vi "Unflatten Pixmap.vi"(10 "image data":T1) -> (0 "1-bit pixmap":bool[][](array[boolean]), 1 "4-bit pixmap":u8[][](array[numeric]), 2 "8-bit pixmap":u8[][](array[numeric]), 3 "24-bit pixmap":u32[][](array[numeric]) format="%x", 4 "colors":u32[](array[numeric]), 5 "top left":cluster{"x":i16, "y":i16}, 6 "mask":u8[](array[numeric]))   [LabVIEW 2017]
doc: "Converts a cluster of image data into a 2D array."
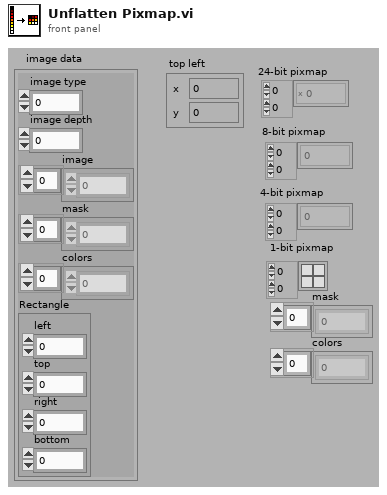
[diagram p1: front panel]
types:
  T1 = cluster{"image type":i32, "image depth":i32, "image":u8[], "mask":u8[], "colors":u32[], "Rectangle":cluster{"left":i16, "top":i16, "right":i16, "bottom":i16}}
  T2 = cluster{"left":i16, "top":i16, "right":i16, "bottom":i16}
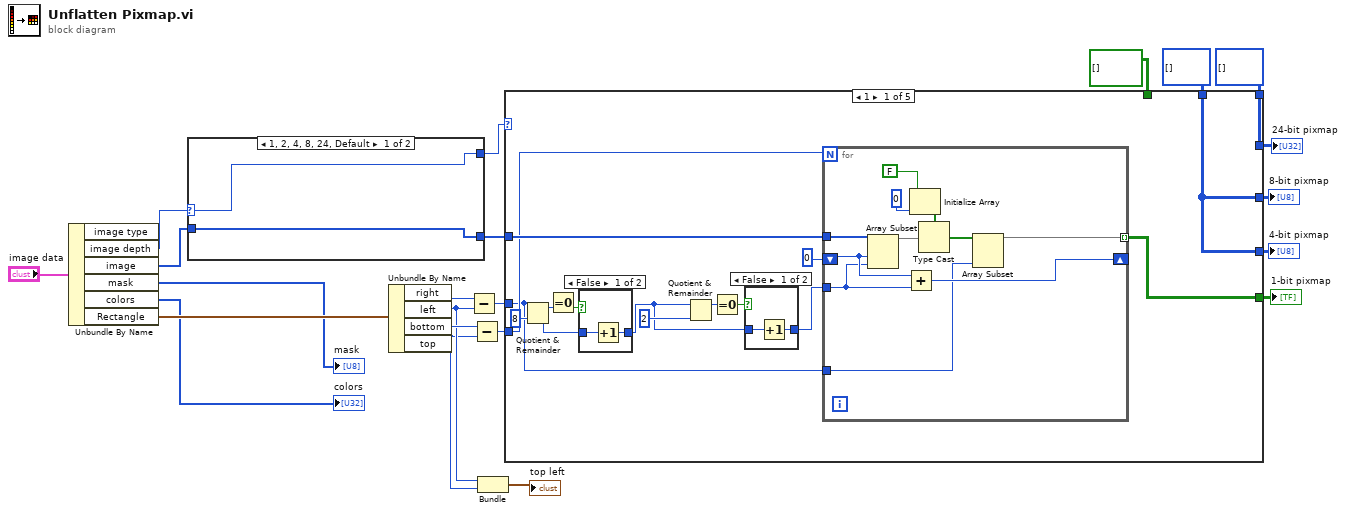
[diagram p0: block diagram]
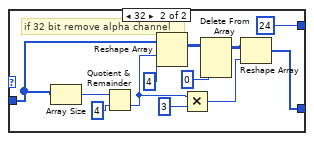
[diagram p2: hidden frame]
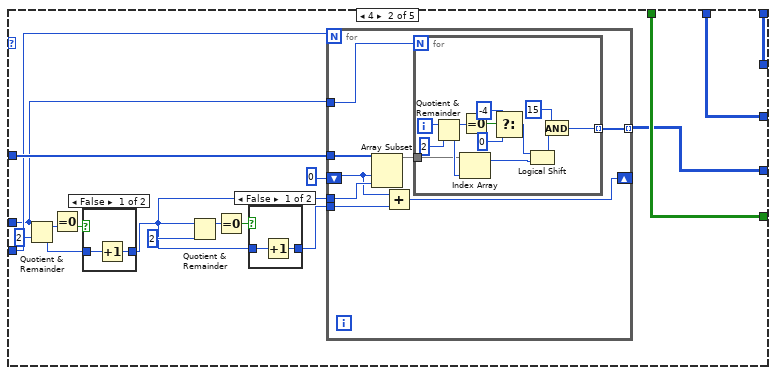
[diagram p5: hidden frame]
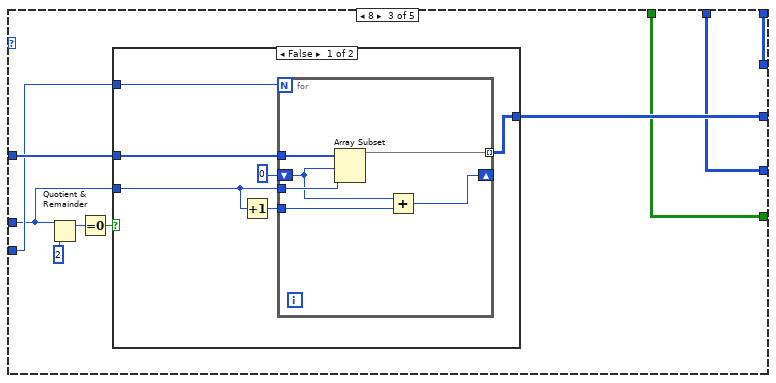
[diagram p8: hidden frame]
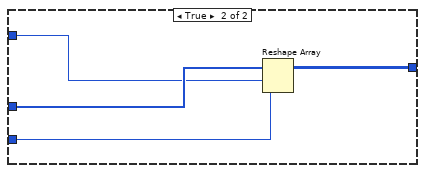
[diagram p9: hidden frame]
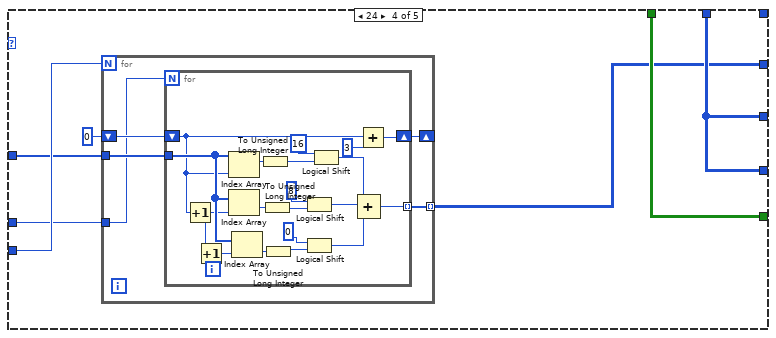
[diagram p10: hidden frame]
diagram:
  n1 = Unbundle By Name("image data") -> ("image depth"=w1:i32, "image"=w4:u8[], "mask"=→"mask":u8[], "colors"=→"colors":u32[], "Rectangle"=w7:T2)  [unwired: 1 out]
  n2 = case shown="1, 2, 4, 8, 24, Default" w1 {
    selector: w1 -> [w24 _]
    tunnel: [w24 24] -> w2
    tunnel: w4 -> [w23 w35]
    tunnel: [w23 w26] -> w3
    frame 1, 2, 4, 8, 24, Default {
    }
    frame 32 {
      # "if 32 bit remove alpha channel"
      n3 = Array Size(array=w35) -> (size(s)=w34:i32)
      n4 = Quotient & Remainder(x=w34, y=4) -> (floor(x/y)=w30:i32)  [unwired: 1 out]
      n5 = Reshape Array(w35, w30, 4 ("dimension size")) -> (w32:u8[][])
      n6 = Multiply(x=w30, y=3) -> (x*y=w28:i32)
      n7 = Delete From Array(array=w32, index (col)=0 ("dimension size")) -> (array with subset deleted=w27:u8[][])  [unwired: 2 in, 1 out]
      n8 = Reshape Array(w27, w28) -> (w26:u8[])
    }
  }
  n9 = Unbundle By Name(w7) -> ("right"=w22:i16, "left"=w10:i16, "bottom"=w21:i16, "top"=w9:i16)
  n10 = Subtract(x=w22, y=w10) -> (x-y=w20:i16)
  n11 = Subtract(x=w21, y=w9) -> (x-y=w19:i16)
  n12 = Bundle("left"=w10, "top"=w9) -> (→"top left":cluster{"left":i16, "top":i16})  [unwired: 1 in]
  n13 = case shown="1" w2 {
    tunnel: w3 -> [w52 w86 w121 w142 _]
    tunnel: w20 -> [w39 w72 w118 w143 _]
    tunnel: w19 -> [w44 w78 w119 w144 _]
    tunnel: [w47 w71 w114 w146 w172] -> w18
    tunnel: u8[][] [] ("4-bit pixmap") -> [w46 w80 w115 w145 w171]
    tunnel: [w46 w70 w115 w145 w171] -> w16
    tunnel: bool[][] [] ("1-bit pixmap") -> [_ w71 w114 w146 w172]
    tunnel: [w46 w80 w120 w145 w171] -> w14
    tunnel: [w45 w79 w116 w141 w173] -> w13
    tunnel: u32[][] [] ("24-bit pixmap") -> [w45 w79 w116 _ w173]
    frame 1 {
      n14 = Quotient & Remainder(x=w39, y=i16 8) -> (x-y*floor(x/y)=w42:i16, floor(x/y)=w40:i16)
      n15 = Equal To 0?(x=w42) -> (x = 0?=w41:bool)
      n16 = case shown="False" w41 {
        tunnel: w40 -> [w54 w55]
        tunnel: [w53 w55] -> w38
        frame False {
          n17 = Increment(x=w54) -> (x+1=w53:i16)
        }
        frame True {
        }
      }
      n18 = Quotient & Remainder(x=w38, y=2) -> (x-y*floor(x/y)=w50:i32)  [unwired: 1 out]
      n19 = Equal To 0?(x=w50) -> (x = 0?=w49:bool)
      n20 = case shown="False" w49 {
        tunnel: w38 -> [w57 w58]
        tunnel: [w56 w58] -> w37
        frame False {
          n21 = Increment(x=w57) -> (x+1=w56:i16)
        }
        frame True {
        }
      }
      n22 = for {
        N: w44 -> [_]
        tunnel: w52 -> [w69]
        shift-right: [w64] -> _
        shift-left: 0 -> [w68]
        tunnel: w37 -> [w59]
        tunnel: [w61] -> w47 mode=indexing
        tunnel: w39 -> [w62]
        n23 = Array Subset(array=w69, index=w68, length=w59) -> (w60:u8[])
        n24 = Add(x=w68, y=w59) -> (x+y=w64:i32)
        n25 = Initialize Array(FALSE, i16 0) -> (w67:bool[])
        n26 = Type Cast(type=w67, x=w60) -> (*(type *) &x=w63:bool[])
        n27 = Array Subset(array=w63, length=w62) -> (w61:bool[])  [unwired: 1 in]
      }
    }
    frame 4 {
      n28 = Quotient & Remainder(x=w72, y=i16 2) -> (x-y*floor(x/y)=w76:i16, floor(x/y)=w74:i16)
      n29 = Equal To 0?(x=w76) -> (x = 0?=w75:bool)
      n30 = case shown="False" w75 {
        tunnel: w74 -> [w88 w89]
        tunnel: [w87 w89] -> w73
        frame False {
          n31 = Increment(x=w88) -> (x+1=w87:i16)
        }
        frame True {
        }
      }
      n32 = Quotient & Remainder(x=w73, y=2) -> (x-y*floor(x/y)=w84:i32)  [unwired: 1 out]
      n33 = Equal To 0?(x=w84) -> (x = 0?=w83:bool)
      n34 = case shown="False" w83 {
        tunnel: w73 -> [w91 w92]
        tunnel: [w90 w92] -> w81
        frame False {
          n35 = Increment(x=w91) -> (x+1=w90:i16)
        }
        frame True {
        }
      }
      n36 = for {
        N: w78 -> [_]
        tunnel: w86 -> [w100]
        shift-right: [w96] -> _
        shift-left: 0 -> [w98]
        tunnel: w73 -> [w99]
        tunnel: w81 -> [w97]
        tunnel: w72 -> [w93]
        tunnel: [w94] -> w70 mode=indexing
        n37 = Array Subset(array=w100, index=w98, length=w99) -> (w95:u8[])
        n38 = Add(x=w98, y=w97) -> (x+y=w96:i32)
        n39 = for {
          N: w93 -> [_]
          tunnel: w95 -> [w107]
          tunnel: [w108] -> w94 mode=indexing
          i -> [w112]
          n40 = Quotient & Remainder(x=w112, y=2) -> (x-y*floor(x/y)=w105:i32, floor(x/y)=w111:i32)
          n41 = Index Array(array=w107, index=w111) -> (element=w106:u8)
          n42 = Equal To 0?(x=w105) -> (x = 0?=w104:bool)
          n43 = Select(t=i8 -4, s=w104, f=i8 0) -> (s? t:f=w101:i8)
          n44 = Logical Shift(y=w101, x=w106) -> (x << y=w109:u8)
          n45 = And(x=u8 15, y=w109) -> (x .and. y?=w108:u8)
        }
      }
    }
    frame 8 {
      n46 = Quotient & Remainder(x=w118, y=2) -> (x-y*floor(x/y)=w122:i32)  [unwired: 1 out]
      n47 = Equal To 0?(x=w122) -> (x = 0?=w117:bool)
      n48 = case shown="False" w117 {
        tunnel: w121 -> [w129 w138]
        tunnel: [w126 w139] -> w120
        tunnel: w119 -> [w128 w137]
        tunnel: w118 -> [w125 w136]
        frame False {
          n49 = Increment(x=w125) -> (x+1=w124:i16)
          n50 = for {
            N: w128 -> [_]
            tunnel: w129 -> [w135]
            shift-right: [w132] -> _
            shift-left: 0 -> [w133]
            tunnel: w125 -> [w134]
            tunnel: [w131] -> w126 mode=indexing
            tunnel: w124 -> [w130]
            n51 = Array Subset(array=w135, index=w133, length=w134) -> (w131:u8[])
            n52 = Add(x=w133, y=w130) -> (x+y=w132:i32)
          }
        }
        frame True {
          n53 = Reshape Array(w138, w137, w136) -> (w139:u8[][])
        }
      }
    }
    frame 24 {
      n54 = for {
        N: w144 -> [_]
        tunnel: w143 -> [w147]
        tunnel: w142 -> [w151]
        tunnel: [w150] -> w141 mode=indexing
        shift-right: [w148] -> _
        shift-left: 0 -> [w149]
        n55 = for {
          N: w147 -> [_]
          tunnel: w151 -> [w170]
          tunnel: [w160] -> w150 mode=indexing
          shift-right: [w158] -> w148
          shift-left: w149 -> [w157]
          n56 = Increment(x=w157) -> (x+1=w156:i32)
          n57 = Increment(x=w156) -> (x+1=w169:i32)
          n58 = Index Array(array=w170, index=w157) -> (element=w163:u8)
          n59 = Index Array(array=w170, index=w156) -> (element=w155:u8)
          n60 = Index Array(array=w170, index=w169) -> (element=w164:u8)
          n61 = To Unsigned Long Integer(number=w163) -> (unsigned 32bit integer=w153:u32)
          n62 = To Unsigned Long Integer(number=w155) -> (unsigned 32bit integer=w166:u32)
          n63 = To Unsigned Long Integer(number=w164) -> (unsigned 32bit integer=w165:u32)
          n64 = Logical Shift(y=i8 8, x=w166) -> (x << y=w162:u32)
          n65 = Logical Shift(y=i8 0, x=w165) -> (x << y=w161:u32)
          n66 = Logical Shift(y=i8 16, x=w153) -> (x << y=w152:u32)
          n67 = Add(x=w157, y=3) -> (x+y=w158:i32)
          n68 = Compound Arithmetic op=ADD(w152, w162, w161) -> (w160:u32)
        }
      }
    }
    frame Default {
    }
  }
  "1-bit pixmap" <- w18
  "4-bit pixmap" <- w16
  "8-bit pixmap" <- w14
  "24-bit pixmap" <- w13
